vi "AbortMeasurement.vi"(7 "error in (no error)":errorcluster) -> (0 "error out":errorcluster)   [LabVIEW 2015, in "ESLSCDLL.lvlib"]
uses:
  ESLSCDLL.lvlib
  Globals.vi
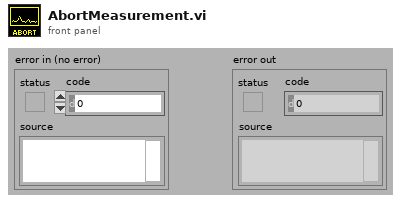
[diagram p1: front panel]
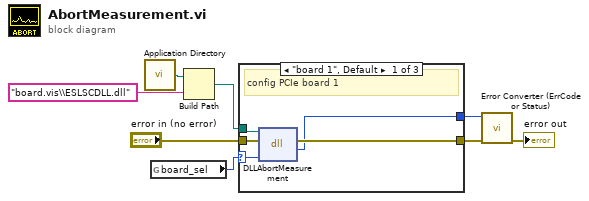
[diagram p0: block diagram]
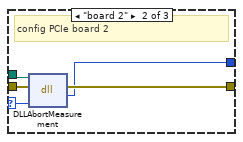
[diagram p2: hidden frame]
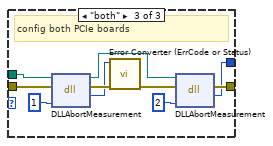
[diagram p3: hidden frame]
diagram:
  n1 = call <vilib>:"Application Directory.vi"() -> ("Application Directory"=w3:path)
  n2 = global read "Globals.vi" "board_sel"() -> (w4:enum32{"0", "board 1", "board 2", "both"})
  n3 = Build Path(base path=w3, name or relative path="board.vis\\ESLSCDLL.dll") -> (appended path=w1:path)
  n4 = case shown="\"board 1\", Default" w4 {
    selector: w4 -> [w13 w18 _]
    tunnel: "error in (no error)" -> [w12 w17 w26]
    tunnel: [w11 w16 w22] -> w7
    tunnel: [w10 w15 w21] -> w5
    tunnel: w1 -> [w9 w14 w20]
    frame "board 1", Default {
      # "config PCIe board 1"
      n5 = dll-call lib="C:/ENTW/PCIE/LV64/board.vis/ESLSCDLL.dll" fn="DLLAbortMeasurement" ("lwlscdll.dll:DLLOpenShutter")(path in=w9, error in=w12, "drv"=w13) -> (error out=w11:errorcluster, "es_status_codes"=w10:i32)  [unwired: 2 in, 1 out]
    }
    frame "board 2" {
      # "config PCIe board 2"
      n6 = dll-call lib="C:/ENTW/PCIE/LV64/board.vis/ESLSCDLL.dll" fn="DLLAbortMeasurement" ("lwlscdll.dll:DLLOpenShutter")(path in=w14, error in=w17, "drv"=w18) -> (error out=w16:errorcluster, "es_status_codes"=w15:i32)  [unwired: 2 in, 1 out]
    }
    frame "both" {
      # "config both PCIe boards"
      n7 = dll-call lib="C:/ENTW/PCIE/LV64/board.vis/ESLSCDLL.dll" fn="DLLAbortMeasurement" ("lwlscdll.dll:DLLOpenShutter")(path in=w20, error in=w26, "drv"=u32 1) -> (path out=w19:path, error out=w25:errorcluster, "es_status_codes"=w24:i32)  [unwired: 2 in]
      n8 = call "Error Converter (ErrCode or Status).vi"("error in (no error)"=w25, "error code"=w24) -> ("error out"=w23:errorcluster)  [unwired: 9 in]
      n9 = dll-call lib="C:/ENTW/PCIE/LV64/board.vis/ESLSCDLL.dll" fn="DLLAbortMeasurement" ("lwlscdll.dll:DLLOpenShutter")(path in=w19, error in=w23, "drv"=u32 2) -> (error out=w22:errorcluster, "es_status_codes"=w21:i32)  [unwired: 2 in, 1 out]
    }
  }
  n10 = call "Error Converter (ErrCode or Status).vi"("error in (no error)"=w7, "error code"=w5) -> ("error out"=→"error out":errorcluster)  [unwired: 9 in]
